vi "PS Control Launcher.vi"() -> ()   [LabVIEW 2020]
uses:
  PS Driver/AMI 4xx/PS Driver AMI4xx.lvclass
  Users/sth/Documents/Winders Shared Folders/Winders LV 20/NML Data Acquisition LV20/SCM PS Actor Framework/PS Driver/PS Driver.lvclass
  PS Control Actor.lvclass
  PS Control Persistence Actor/PS Control Persistence Actor.lvclass
  Users/sth/Documents/Winders Shared Folders/Winders LV 20/NML Data Acquisition LV20/SCM PS Actor Framework/PS Control Actor/PS Control Actor.lvclass
panel:
  in  "stop":bool
  out "error out":errorcluster
  # "Starting PS Control"
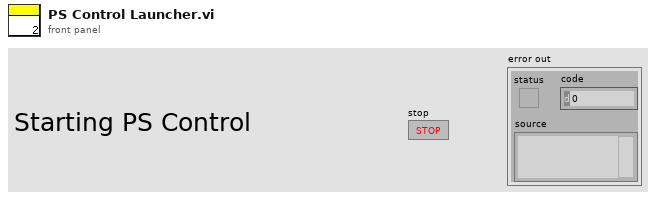
[diagram p1: front panel]
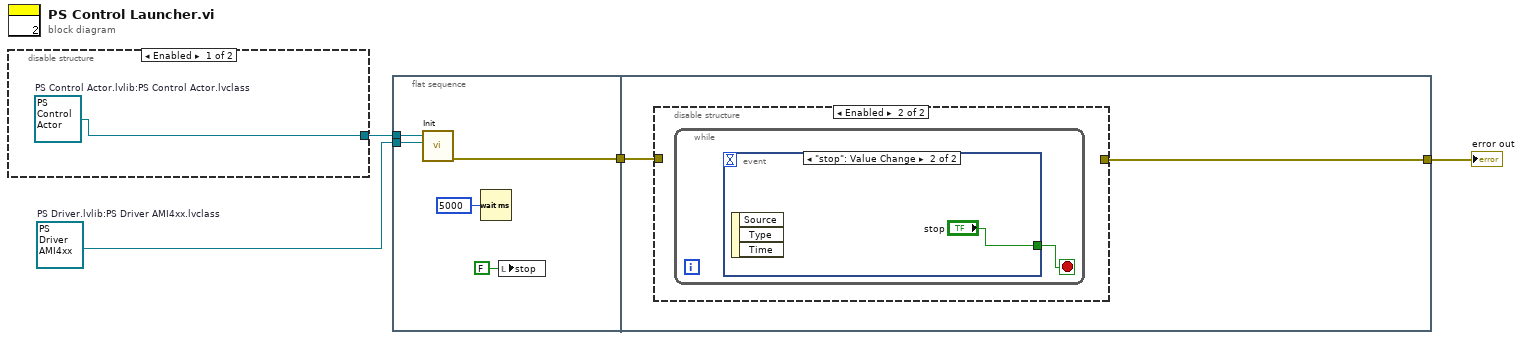
[diagram p0: block diagram]
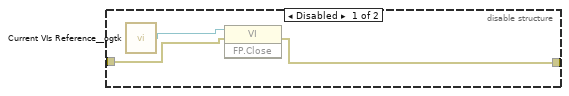
[diagram p2: hidden frame]
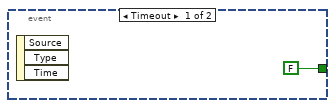
[diagram p3: hidden frame]
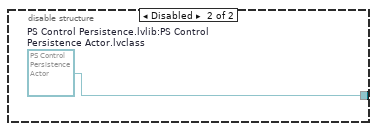
[diagram p4: hidden frame]
diagram:
  w3 = refnum<class "PS Driver AMI4xx.lvclass"> refnum  # PS Driver.lvlib:PS Driver AMI4xx.lvclass
  n1 = disable-structure shown="Enabled" {
    disable-tunnel: [w5 w6] -> w4
    frame Enabled {
      w5 = refnum<class "PS Control Actor.lvclass"> refnum  # PS Control Actor.lvlib:PS Control Actor.lvclass
    }
    frame Disabled {
      w6 = refnum<class "PS Control Persistence Actor.lvclass"> refnum  # PS Control Persistence.lvlib:PS Control Persistence Actor.lvclass
    }
  }
  n2 = flat-sequence {
    tunnel: w4 -> [w11]
    tunnel: w3 -> [w10]
    tunnel: [w8] -> w2
    tunnel: w2 -> [w13]
    tunnel: [w12] -> w1
    frame #0 {
      n3 = call "Init.vi"("PS Driver.lvlib:PS Driver.lvclass"=w10, "PS Control Actor in"=w11) -> ("error out"=w8:errorcluster)  [unwired: 8 in, 1 out]
      n4 = Wait (ms)(milliseconds to wait=u32 5000) -> ()  [unwired: 1 out]
      n5 = local write "stop"(FALSE ("stop")) -> ()
    }
    frame #1 {
      n6 = disable-structure shown="Enabled" {
        disable-tunnel: w13 -> [w15 _]
        disable-tunnel: [w14 _] -> w12
        frame Disabled {
          n7 = call <userlib>:"Current VIs Reference__ogtk.vi"() -> ("Current VI's reference"=w16:refnum<vi>)  [unwired: 5 in]
          n8 = invoke class="VI" method="FP.Close"(reference=w16, error in=w15) -> (error out=w14:errorcluster)  [unwired: 1 in, 2 out]
        }
        frame Enabled {
          n9 = while {
            stop <- w17 stop-if-true
            n10 = event shown="[1] \"stop\": Value Change" {
              selector: _ -> [_ _]
              dyn-events: _ -> [_ _]
              timeout: _ -> [_ _]
              tunnel: [FALSE "stop"] -> w17
              event Timeout {
                n11 = event-data() -> ()  [unwired: 1 in, 3 out]
              }
              event "stop": Value Change {
                n12 = event-data() -> ()  [unwired: 1 in, 3 out]
              }
            }
          }
        }
      }
    }
  }
  "error out" <- w1
